vi "Agilent 3446X Series Acquire Single.vi"() -> ()   [LabVIEW 2021]
doc: "This example shows how to configure a measurement and take a reading."
uses:
  <instrlib>/Agilent 3446X Series/Public/Data/Read (Single Point).vi
  <instrlib>/Agilent 3446X Series/Agilent 3446X Series.lvlib
panel:
  in  "error in":errorcluster
  out "error out":errorcluster
  in  "Measurement Function":i32(ring)=10 items=["Continuity", "Current AC", "Current DC", "Diode", "Frequency", "Resistance 4-wire", "Period", "Resistance 2-wire", "Temperature", "Voltage AC", "Voltage DC", "Voltage DC Ratio", "Capacitance"]
  in  "Absolute Resolution":dbl=1e-06
  in  "Agilent DMM":refnum<visa-resource-name>
  in  "Manual Range (1)":dbl=1.0
  out "Measurement":dbl
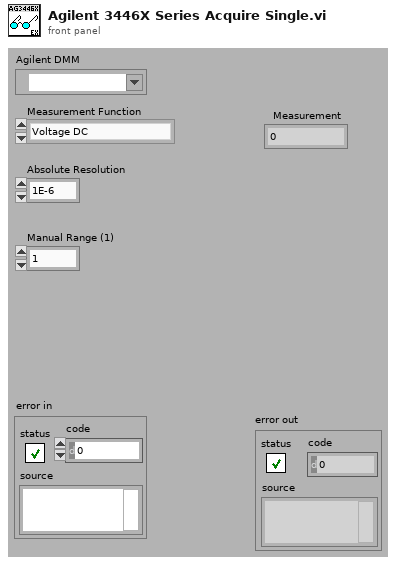
[diagram p1: front panel]
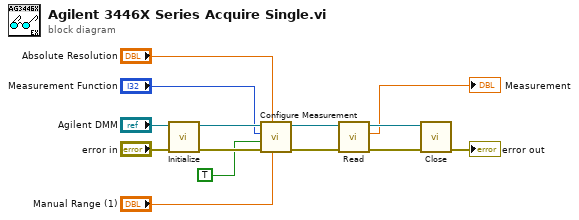
[diagram p0: block diagram]
diagram:
  n1 = call <instrlib>:"Initialize.vi"("error in (no error)"="error in", "VISA resource name"="Agilent DMM") -> ("error out"=w13:errorcluster, "VISA resource name out"=w14:refnum<visa-resource-name>)  [unwired: 3 in, 5 out]
  n2 = call <instrlib>:"Configure Measurement.vi"("Manual Range (1)"="Manual Range (1)", "Absolute Resolution (1E-6)"="Absolute Resolution", "error in (no error)"=w13, "Auto Range (T: Enable)"=TRUE, "Measurement Function (10: Voltage DC)"="Measurement Function", "VISA resource name"=w14) -> ("error out"=w9:errorcluster, "VISA resource name out"=w10:refnum<visa-resource-name>)  [unwired: 4 out]
  n3 = call-poly <instrlib>:"Read.vi"("error in (no error)"=w9, "VISA resource name"=w10) -> ("error out"=w12:errorcluster, "Measurement"=→"Measurement":dbl, "VISA resource name out"=w11:refnum<visa-resource-name>)  [unwired: 7 out]
  n4 = call <instrlib>:"Close.vi"("error in (no error)"=w12, "VISA resource name"=w11) -> ("error out"=→"error out":errorcluster)  [unwired: 9 out]
